vi "svfa_Check Data Valid [Dual FFT subset].vi"(0 "stimulus [X]":waveform(dbl)={"t0"=timestamp(0 s since 1904-01-01), "dt"=1.953125e-05, "Y"=[]}, 1 "response [Y]":waveform(dbl)={"t0"=timestamp(0 s since 1904-01-01), "dt"=1.953125e-05, "Y"=[]}, 2 "window":T3 items=["None "=0, "Hanning"=1, "Hamming"=2, "Blackman-Harris"=3, "Exact Blackman"=4, "Blackman"=5, "Flat Top"=6, "4 Term B-Harris "=7, "7 Term B-Harris"=8, "Low Sidelobe"=9, "Force - Exponential"=10, "Gaussian"=11, "<30>"=30, "<31>"=31, "<32>"=32, "<33>"=33, "<34>"=34, "<60>"=60, "<61>"=61, "<62>"=62], 3 "force/exp settings":T2={"force window [%]"=50.0, "exp window [%]"=10.0} {"exp window [%]" min=0.0 max=100.0 format="%.2f"; "force window [%]" min=0.0 max=100.0 format="%.2f"}, 4 "averaging parameters":T5={"averaging mode"=enum."No averaging", "weighting mode"=enum."Linear", "number of averages"=10, "linear mode"=enum."Auto restart"}, 5 "error in (no error)":errorcluster, 6 "frequency range":T6={"start frequency"=20.0, "stop frequency"=20000.0} {"stop frequency" format="%.2f"; "start frequency" format="%.2f"}, 7 "processing control in":T4(ring), 8 "restart averaging (F)":bool, 9 "FRF mode":enum16{"H1", "H2", "H3"}(ring), 10 "measurement":T1(ring)=enum."Frequency response") -> (11 "dup FRF mode":enum16{"H1", "H2", "H3"}(ring), 12 "dup frequency range":T6={"start frequency"=20.0, "stop frequency"=20000.0} {"stop frequency" format="%.2f"; "start frequency" format="%.2f"}, 13 "processing control out":T4(ring), 14 "dup stimulus [X]":waveform(dbl)={"t0"=timestamp(0 s since 1904-01-01), "dt"=1.953125e-05, "Y"=[]}, 15 "dup response [Y]":waveform(dbl)={"t0"=timestamp(0 s since 1904-01-01), "dt"=1.953125e-05, "Y"=[]}, 16 "window":u16(ring) items=["None "=0, "Hanning"=1, "Hamming"=2, "Blackman-Harris"=3, "Exact Blackman"=4, "Blackman"=5, "Flat Top"=6, "4 Term B-Harris "=7, "7 Term B-Harris"=8, "Low Sidelobe"=9, "Force - Exponential"=10, "Gaussian"=62], 17 "dup force/exp settings":T2={"force window [%]"=50.0, "exp window [%]"=10.0} {"exp window [%]" min=0.0 max=100.0 format="%.2f"; "force window [%]" min=0.0 max=100.0 format="%.2f"}, 18 "dup averaging parameters":T5={"averaging mode"=enum."No averaging", "weighting mode"=enum."Linear", "number of averages"=10, "linear mode"=enum."Auto restart"}, 19 "error out":errorcluster)   [LabVIEW 2017]
uses:
  <vilib>/addons/_NISVFA/_Shared subVIs/Controls/svc_Window [Dual FFT].ctl
  <vilib>/addons/_NISVFA/_Shared subVIs/Common/svc_Check for Waveform Parameter Continuity (1 Ch).vi
  <vilib>/addons/_NISVFA/_Shared subVIs/Common/svc_Check for Waveform Parameter Continuity (no state).vi
  <vilib>/addons/_NISVFA/_Shared subVIs/Common/svc_Get SV Channel Info.vi
  <vilib>/addons/_NISVFA/_Shared subVIs/Common/svc_Check dt for Equal Sample Rates.vi
  <vilib>/addons/_NISVFA/_Shared subVIs/Common/svc_Engineering Units to Unit Label.vi
  <vilib>/addons/_NISVFA/_Shared subVIs/Common/svc_Unit Label to Engineering Units.vi
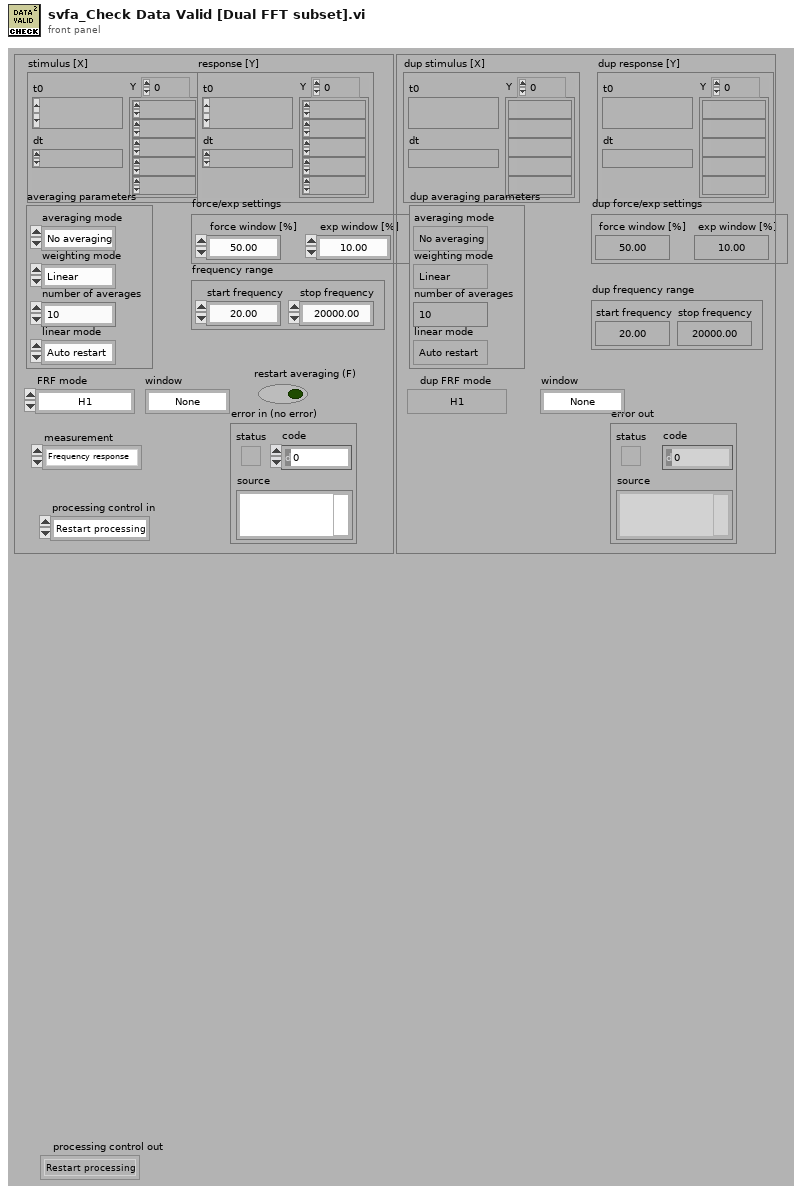
[diagram p1: front panel]
types:
  T1 = enum16{"Cross spectrum", "Frequency response", "Coherent output power"}
  T2 = cluster{"force window [%]":dbl, "exp window [%]":dbl}
  T3 = typedef "svc_Window [Dual FFT].ctl" = u32
  T4 = enum16{"Restart processing", "Continue processing", "Skip processing"}
  T5 = cluster{"averaging mode":enum16{"No averaging", "Vector averaging", "RMS averaging", "Peak hold"}, "weighting mode":enum16{"Linear", "Exponential"}, "number of averages":u32, "linear mode":enum16{"One shot", "Auto restart"}}
  T6 = cluster{"start frequency":dbl, "stop frequency":dbl}
  T7 = cluster{"dt":bool, "t0 continuity":bool, "array length":bool, "channel info":bool, "name":bool}
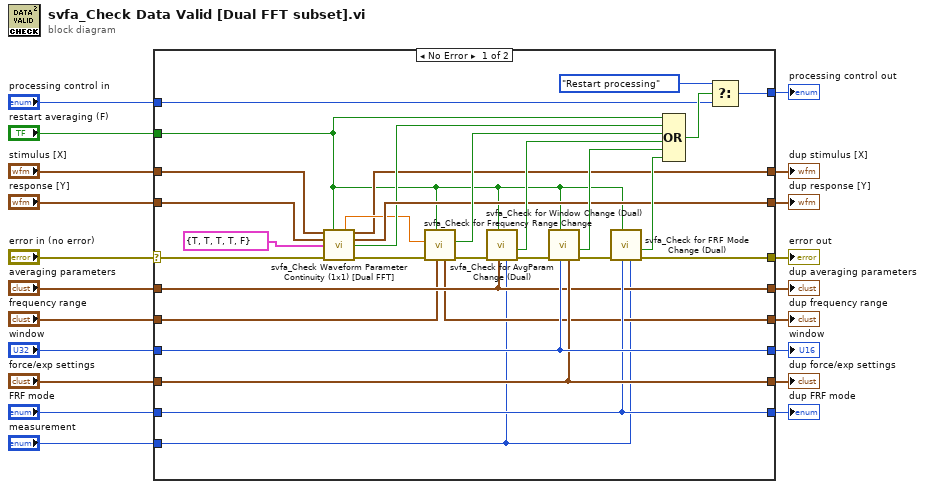
[diagram p0: block diagram]
diagram:
  n1 = case shown="No Error" "error in (no error)" {
    selector: "error in (no error)" -> [w23 w58]
    tunnel: [w21 w58] -> w20
    tunnel: "stimulus [X]" -> [w31 w57]
    tunnel: [w24 w57] -> w18
    tunnel: "response [Y]" -> [w30 w56]
    tunnel: [w29 w56] -> w16
    tunnel: "restart averaging (F)" -> [w22 _]
    tunnel: "frequency range" -> [w39 w55]
    tunnel: [w40 w55] -> w12
    tunnel: "window" -> [w49 w54]
    tunnel: [w49 w54] -> w10
    tunnel: [w46 w53] -> w8
    tunnel: "FRF mode" -> [w46 w53]
    tunnel: "force/exp settings" -> [w48 w52]
    tunnel: [w48 w52] -> w6
    tunnel: "averaging parameters" -> [w41 w51]
    tunnel: [w41 w51] -> w4
    tunnel: "processing control in" -> [w43 w50]
    tunnel: [w42 w50] -> w2
    tunnel: "measurement" -> [w38 _]
    frame No Error {
      n2 = call <vilib>:"svfa_Check Waveform Parameter Continuity (1x1) [Dual FFT].vi"("stimulus signal X [EUx]"=w31, "restart averaging (F)"=w22, "response signal Y [EUy]"=w30, "checks for channel parameter change"=T7 {"dt"=TRUE, "t0 continuity"=TRUE, "array length"=TRUE, "channel info"=TRUE, "name"=FALSE}, "error in"=w23) -> ("dt"=w25:dbl, "stimulus signal X [EUx]"=w24:waveform(dbl), "response signal Y [EUy]"=w29:waveform(dbl), "waveform parameter changed"=w26:bool, "error out"=w28:errorcluster)  [unwired: 5 in, 1 out]
      n3 = call <vilib>:"svfa_Check for Frequency Range Change.vi"("frequency range in"=w39, "restart averaging (F)"=w22, "error in (no error)"=w28, "dt"=w25) -> ("error out"=w36:errorcluster, "Param_has_changed"=w33:bool, "frequency range out"=w40:T6)  [unwired: 5 in]
      n4 = call <vilib>:"svfa_Check for AvgParam Change (Dual).vi"("measurement"=w38, "averaging parameters"=w41, "restart averaging (F)"=w22, "error in (no error)"=w36) -> ("error out"=w35:errorcluster, "parameter has changed"=w34:bool)  [unwired: 6 in]
      n5 = call <vilib>:"svfa_Check for Window Change (Dual).vi"("force/exp settings"=w48, "window"=w49, "restart averaging (F)"=w22, "error in (no error)"=w35) -> ("error out"=w47:errorcluster, "parameter has changed"=w32:bool)  [unwired: 6 in]
      n6 = call <vilib>:"svfa_Check for FRF Mode Change (Dual).vi"("measurement"=w38, "FRF mode"=w46, "restart"=w22, "error in (no error)"=w47) -> ("error out"=w21:errorcluster, "parameter has changed"=w37:bool)  [unwired: 6 in]
      n7 = Compound Arithmetic op=OR(w22, w26, w33, w34, w32, w37) -> (w44:bool)
      n8 = Select(t=T4."Restart processing", s=w44, f=w43) -> (s? t:f=w42:T4)
    }
    frame Error {
    }
  }
  "dup stimulus [X]" <- w18
  "error out" <- w20
  "dup response [Y]" <- w16
  "dup averaging parameters" <- w4
  "dup frequency range" <- w12
  "processing control out" <- w2
  "dup force/exp settings" <- w6
  "dup FRF mode" <- w8
  "window" <- w10
